vi "CSMOMgr-Duplication Check.vi"(8 "Error In":errorcluster caption="error in (no error)", 10 "Queue Name":string, 11 "CSMOMgr":T1) -> (0 "error out":errorcluster, 3 "CSMOMgr Out":T1)   [LabVIEW 2017, in "Communicable State Machine.lvlib"]
uses:
  Communicable State Machine.lvlib
  Def-CSMOMgr.ctl
  CSMQ/_CSMObj.ctl
  CSMQ/_CSMObj-Info.ctl
  Typedef/_CSM_MODE.ctl
  CSMQ/_CSMObj-Refs.ctl
  CSMQ/_CSMObj-Data.ctl
  Priority Queue/Priority Queue.ctl
  Typedef/_Cross CSM State Data.ctl
  Typedef/_CSM_MSG_TYPE.ctl
  Typedef/_Cross CSM State Response.ctl
  Typedef/_CSM_Response Source Message.ctl
  Priority Queue/def-Data(LowPRI-Q).ctl
  CSMQ/_CSMObj-ModeData.ctl
  Typedef/_CSM Status Change Event Data.ctl
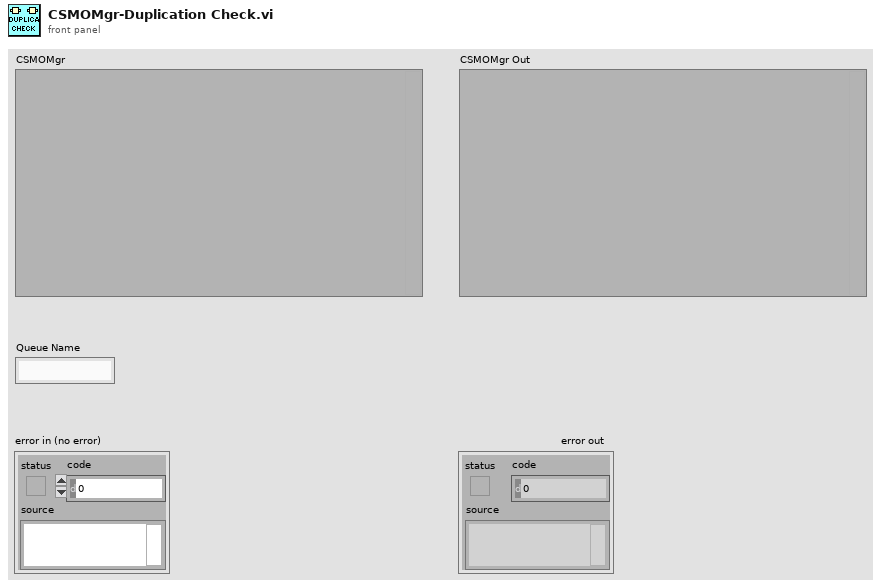
[diagram p1: front panel]
types:
  T1 = typedef "Communicable State Machine.lvlib/Def-CSMOMgr.ctl" = variant
  T2 = typedef "Communicable State Machine.lvlib/_CSMObj.ctl" = cluster{"info":T3, "Refs":T5}
  T3 = typedef "Communicable State Machine.lvlib/_CSMObj-Info.ctl" = cluster{"Module Name":string, "Requested Name":string, "Group Name":string, "Mode":T4, "Allowed Messages":string[]}
  T4 = typedef "Communicable State Machine.lvlib/_CSM_MODE.ctl" = enum16{"Not Exist", "Stand Alone", "CSM", "Worker", "Worker Agent", "Chain Node", "Chain"}
  T5 = typedef "Communicable State Machine.lvlib/_CSMObj-Refs.ctl" = cluster{"WatchDogQ":refnum<queue>, "CSMDataDVR":refnum<data-value>, "Queue":T6, "GroupDataDVR":refnum<data-value>, "TagMap":refnum<data-value>, "ExitEvent":refnum<user-event>, "NewStateEvent":refnum<user-event>, "StatusEvent":refnum<user-event>, "InterruptEvent":refnum<user-event>}
  T6 = typedef "Communicable State Machine.lvlib/Priority Queue.ctl" = cluster{"HPriorityQ":refnum<queue>, "LowPriorityQ":refnum<queue>}
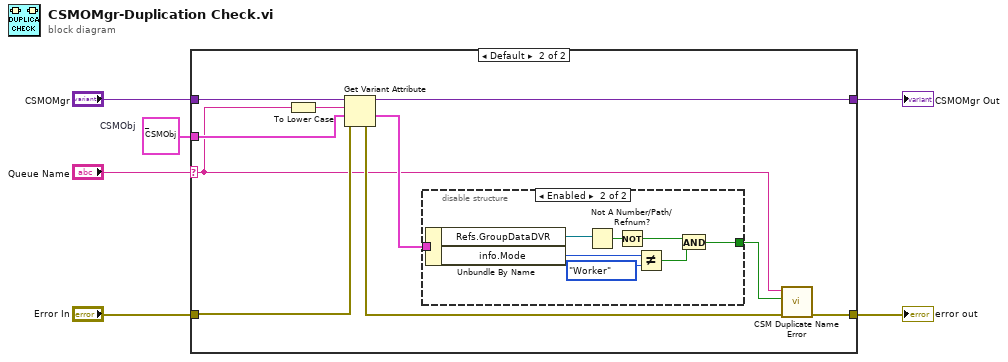
[diagram p0: block diagram]
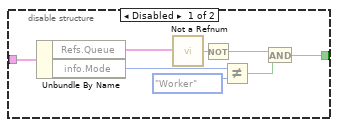
[diagram p3: hidden frame]
diagram:
  w1 = T2 {"info"={"Module Name"="", "Requested Name"="", "Group Name"="", "Mode"=enum."Stand Alone", "Allowed Messages"=[]}, "Refs"={"WatchDogQ"=refnum, "CSMDataDVR"=refnum, "Queue"={"HPriorityQ"=refnum, "LowPriorityQ"=refnum}, "GroupDataDVR"=refnum, "TagMap"=refnum, "ExitEvent"=refnum, "NewStateEvent"=refnum, "StatusEvent"=refnum, "InterruptEvent"=refnum}}  # CSMObj
  n1 = case shown="Default" "Queue Name" {
    selector: "Queue Name" -> [_ w10]
    tunnel: [w7 w18] -> w3
    tunnel: "Error In" -> [w7 w13]
    tunnel: "CSMOMgr" -> [w8 w15]
    tunnel: [w8 w14] -> w2
    tunnel: w1 -> [_ w11]
    frame "", "PostMessageAPI", "SendMessageAPI" {
    }
    frame Default {
      n2 = To Lower Case(string=w10) -> (all lower case string=w9:string)
      n3 = Get Variant Attribute(Variant=w15, name=w9, default value (empty Variant)=w11, error in=w13) -> (duplicate Variant=w14:variant, value=w17:T2, error out=w12:errorcluster)  [unwired: 1 out]
      n4 = disable-structure shown="Enabled" {
        disable-tunnel: w17 -> [w20 w28]
        disable-tunnel: [w19 w27] -> w16
        frame Disabled {
          n5 = Unbundle By Name(w20) -> ("Refs.Queue"=w21:T6, "info.Mode"=w24:T4)
          n6 = call "Not a Refnum.vi"("Priority Queue.lvclass"=w21) -> ("NaN/Path/Refnum?"=w22:bool)  [unwired: 4 in]
          n7 = Not(x=w22) -> (.not. x?=w23:bool)
          n8 = Not Equal?(x=w24, y=_CSM_MODE."Worker") -> (x != y?=w26:bool)
          n9 = And(x=w23, y=w26) -> (x .and. y?=w19:bool)
        }
        frame Enabled {
          n10 = Unbundle By Name(w28) -> ("Refs.GroupDataDVR"=w29:refnum<data-value>, "info.Mode"=w32:T4)
          n11 = Not A Number/Path/Refnum?(number/path/refnum=w29) -> (NaN/Path/Refnum?=w30:bool)
          n12 = Not(x=w30) -> (.not. x?=w31:bool)
          n13 = Not Equal?(x=w32, y=_CSM_MODE."Worker") -> (x != y?=w34:bool)
          n14 = And(x=w31, y=w34) -> (x .and. y?=w27:bool)
        }
      }
      n15 = call "CSM Duplicate Name Error.vi"("error in (no error)"=w12, "Occured"=w16, "CSM Name"=w10) -> ("error out"=w18:errorcluster)  [unwired: 8 in]
    }
  }
  "error out" <- w3
  "CSMOMgr Out" <- w2
